vi "poll_and_write_LiCor_data.vi"(0 "LiCor session in":T2={"VISA resource out"="COM12", "error out"={"status"=FALSE, "code"=0, "source"=""}}, 1 "write to file?":bool, 2 "file session in":T1) -> (4 "CO2 integral":dbl, 5 "LiCor session out":T2={"VISA resource out"="COM12", "error out"={"status"=FALSE, "code"=0, "source"=""}}, 6 "file session out":T1, 7 "pCO2":dbl)   [LabVIEW 2010]
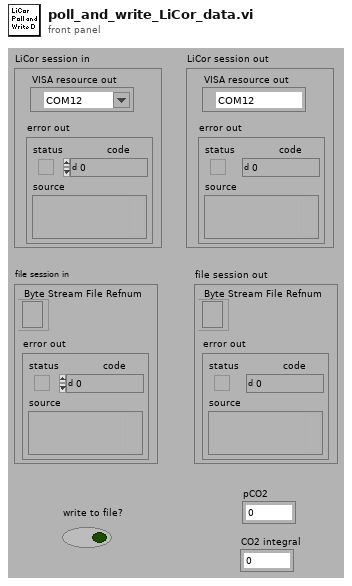
[diagram p1: front panel]
types:
  T1 = cluster{"Byte Stream File Refnum":refnum<file>, "error out":errorcluster}
  T2 = cluster{"VISA resource out":refnum<visa-resource-name>, "error out":errorcluster}
  T3 = cluster{"refnum out":refnum<file>, "error out":errorcluster}
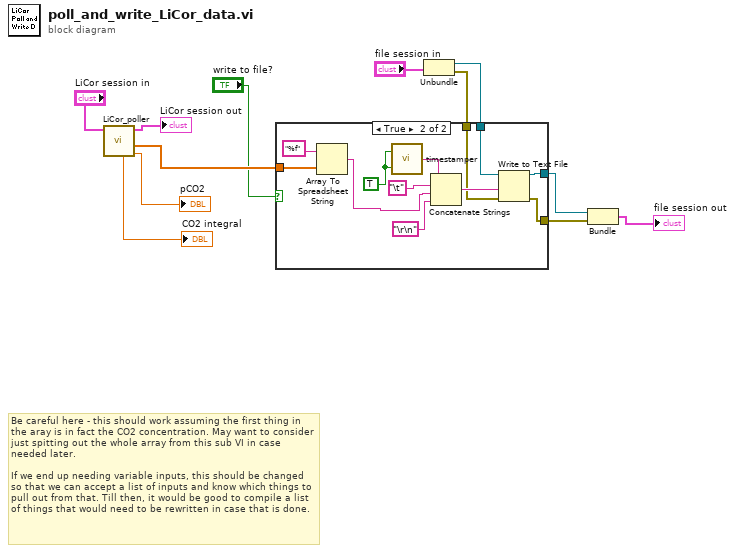
[diagram p0: block diagram]
diagram:
  # "Be careful here - this should work assuming the first thing in the aray is in fact the CO2 concentration. May want to consider just spitting out the whole array from this sub VI in case needed later. \n\nIf we end up needing variable inputs, this should be changed so that we can accept a list of inputs and know which things to pull out from that. Till then, it would be good to compile a list of things that would need to be rewritten in case that is done."
  n1 = call "LiCor_poller.vi"("LiCor session in"="LiCor session in") -> ("pCO2 out"=→"pCO2":dbl, "data array"=w12:dbl[], "LiCor session out"=→"LiCor session out":T2, "Integral out"=→"CO2 integral":dbl)  [unwired: 5 in, 2 out]
  n2 = Unbundle("file session in") -> ("Byte Stream File Refnum"=w7:refnum<file>, "error out"=w6:errorcluster)
  n3 = case shown="True" "write to file?" {
    tunnel: [w14 w25] -> w4
    tunnel: w12 -> [_ w24]
    tunnel: w7 -> [w14 w17]
    tunnel: w6 -> [w13 w16]
    tunnel: [w13 w15] -> w5
    frame False {
    }
    frame True {
      w18 = TRUE
      n4 = Array To Spreadsheet String(array=w24, 3:"%f") -> (spreadsheet string=w23:string)  [unwired: 1 in]
      n5 = call "timestamper.vi"("seconds?"=w18, "ms?"=w18) -> ("datetime output"=w19:string)
      n6 = Concatenate Strings(w19, "\t", w23, "\r\n") -> (w22:string)
      n7 = Write to Text File(file (use dialog)=w17, text=w22, error in=w16) -> (refnum out=w25:refnum<file>, error out=w15:errorcluster)  [unwired: 1 in, 1 out]
    }
  }
  n8 = Bundle("refnum out"=w4, "error out"=w5) -> (→"file session out":T3)  [unwired: 1 in]
